vi "Build Events Summary.vi"(8 "error in (no error)":errorcluster, 11 "Event Reporter Module in":refnum<class "Event Reporter Module.lvclass">) -> (0 "error out":errorcluster, 2 "Events Summary":T1, 3 "Event Reporter Module out":refnum<class "Event Reporter Module.lvclass">)   [LabVIEW 2020, in "Volatus.lvlib" / "Event Reporter Module.lvclass"]
uses:
  Event Reporter Module.lvclass
  Event Reporter Module.lvclass/Event Reporter Module.ctl
  <vilib>/Utility/miscctls.llb/LVMapReplaceAction.ctl
  Events Summary.ctl
  Volatus.lvlib
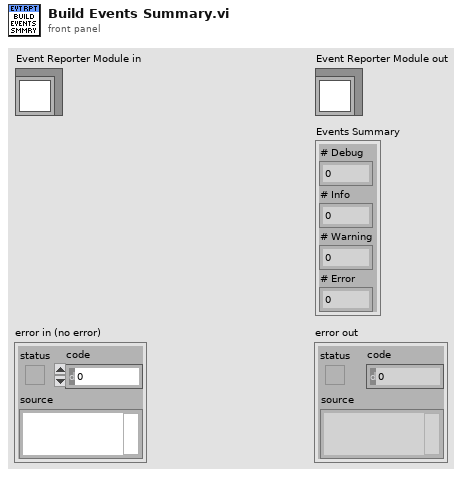
[diagram p1: front panel]
types:
  T1 = typedef "Volatus.lvlib/Events Summary.ctl" = cluster{"# Debug":i32, "# Info":i32, "# Warning":i32, "# Error":i32}
  T2 = typedef "LVMapReplaceAction.ctl" = enum32{"Modify Entry only if found", "Add or Modify Entry", "Delete Entry"}
  T3 = typedef "Volatus.lvlib/Event Reporter Module.lvclass/Event Element.ctl" = cluster{"Node":string, "Node Color":u32, "Timestamp":string, "TS Color":u32, "Level":string, "Level Color":u32, "Context":string, "Context Color":u32, "Message":string, "Error Code":i32, "Error Source":string}
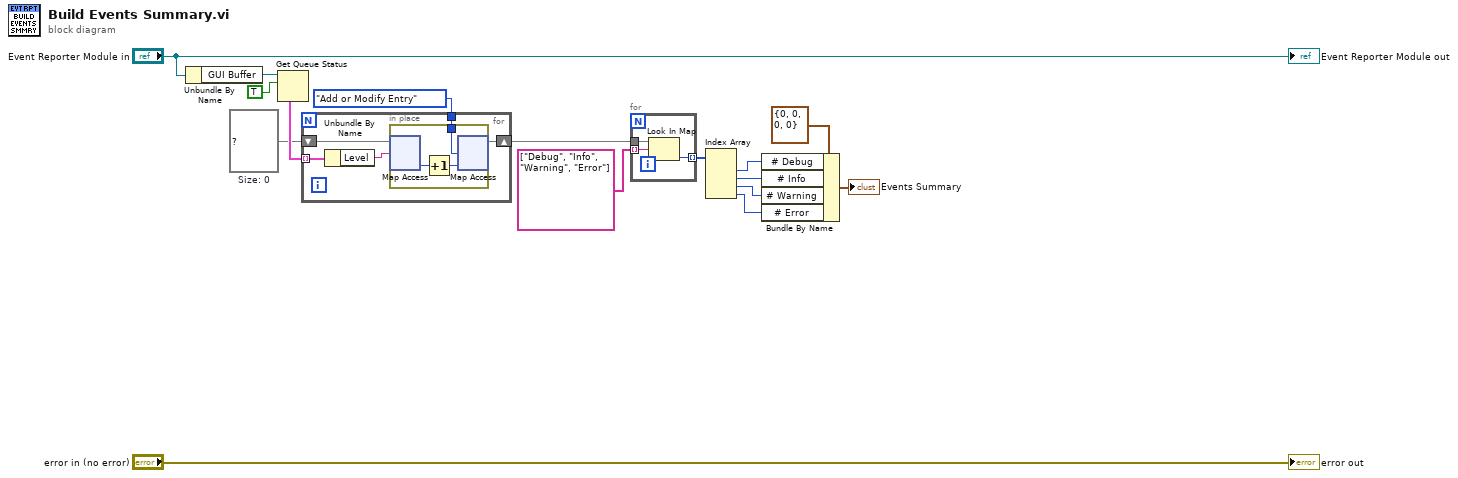
[diagram p0: block diagram]
diagram:
  w12 = map{string, i32} {}  # Size: 0
  n1 = Unbundle By Name("Event Reporter Module in") -> ("GUI Buffer"=w15:refnum<queue>)
  n2 = Get Queue Status(queue=w15, return elements? (F)=TRUE) -> (elements=w13:T3[])  [unwired: 1 in, 7 out]
  n3 = for {
    tunnel: w13 -> [w20] mode=indexing
    shift-right: [w17] -> w9
    shift-left: w12 -> [w21]
    tunnel: LVMapReplaceAction."Add or Modify Entry" ("action") -> [w18]
    n4 = Unbundle By Name(w20) -> ("Level"=w19:string)
    n5 = in-place {
      in-place-border: w18 -> [w22]
      n6 = in-place-map #1(w21, w19) -> (w24:i32)  [unwired: 1 in, 1 out]
      n7 = Increment(x=w24) -> (x+1=w23:i32)
      n8 = in-place-map #1(w23, w22) -> (w17:map{string, i32})  [unwired: 2 out]
    }
  }
  n9 = for {
    tunnel: string[] ["Debug", "Info", "Warning", "Error"] -> [w26] mode=indexing
    tunnel: w9 -> [w27]
    tunnel: [w25] -> w8 mode=indexing
    n10 = Look In Map(map=w27, key=w26) -> (value=w25:i32)  [unwired: 1 in, 1 out]
  }
  n11 = Index Array(array=w8) -> (element #1=w6:i32, element #2=w5:i32, element #3=w4:i32, element #4=w3:i32)  [unwired: 4 in]
  n12 = Bundle By Name(cluster=T1 {"# Debug"=0, "# Info"=0, "# Warning"=0, "# Error"=0} ("Events Summary"), "# Debug"=w6, "# Info"=w5, "# Warning"=w4, "# Error"=w3) -> (→"Events Summary":T1)
  "error out" <- "error in (no error)"
  "Event Reporter Module out" <- "Event Reporter Module in"
